vi "Build SPI Command.vi"(10 "SPI CMD FIFO Element":u64, 11 "SPI PHY Settings":T2={"Divide Value"=20, "Transfer Length (bits)"=32, "CS Asserted Polarity"=FALSE, "Clock Polarity (CPOL)"=FALSE, "Clock Phase (CPHA)"=FALSE, "Lengthen MISO Setup"=FALSE, "Direction Change Bit"=0, "MOSI Starts as Output"=FALSE, "Tristatable MOSI"=FALSE} {"Direction Change Bit" max=64 step=1; "Transfer Length (bits)" min=1 max=64 step=1}) -> (2 "SLSC SPI Command":T1={"Chip Select"=0, "CS Bit Value/Slot #"=0, "SPI PHY Settings"={"Divide Value"=0, "Transfer Length (bits)"=1, "CS Asserted Polarity"=FALSE, "Clock Polarity (CPOL)"=FALSE, "Clock Phase (CPHA)"=FALSE, "Lengthen MISO Setup"=FALSE, "Direction Change Bit"=0, "MOSI Starts as Output"=FALSE, "Tristatable MOSI"=FALSE}, "Data to DAC"=0} {"SPI PHY Settings"."Direction Change Bit" max=64 step=1; "SPI PHY Settings"."Transfer Length (bits)" min=1 max=64 step=1}, 3 "Rack #":u8)   [LabVIEW 2014, in "SLSC FPGA Toolkit.lvlib"]
uses:
  SLSC FPGA Toolkit.lvlib
  <userlib>/_NI SPI IP/FPGA/Controllers/Public/Transfer Settings.ctl
  SLSC SPI Command.ctl
  <userlib>/_NI SPI IP/FPGA/Controllers/NI SPI IP FPGA.lvlib
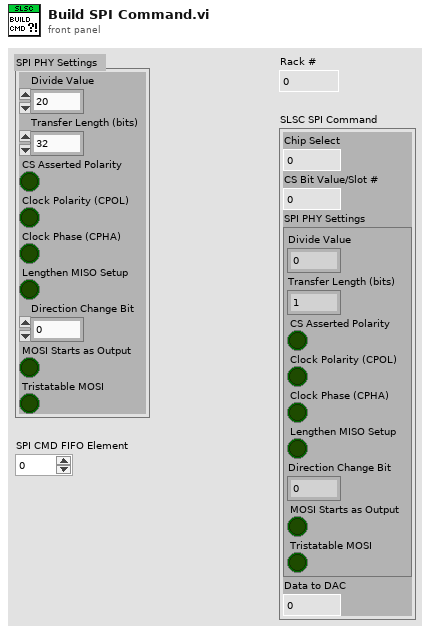
[diagram p1: front panel]
types:
  T1 = typedef "SLSC FPGA Toolkit.lvlib/SLSC SPI Command.ctl" = cluster{"Chip Select":u8, "CS Bit Value/Slot #":u8, "SPI PHY Settings":T2, "Data to DAC":u64}
  T2 = typedef "NI SPI IP FPGA.lvlib/Transfer Settings.ctl" = cluster{"Divide Value":u8, "Transfer Length (bits)":u8, "CS Asserted Polarity":bool, "Clock Polarity (CPOL)":bool, "Clock Phase (CPHA)":bool, "Lengthen MISO Setup":bool, "Direction Change Bit":u8, "MOSI Starts as Output":bool, "Tristatable MOSI":bool}
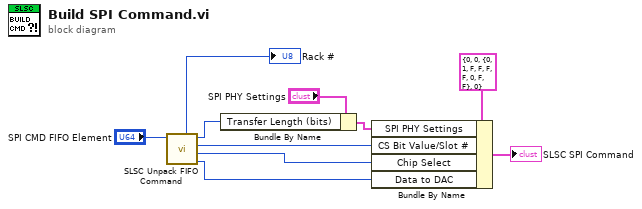
[diagram p0: block diagram]
diagram:
  n1 = call "SLSC Unpack FIFO Command.vi"("SPI CMD FIFO Element"="SPI CMD FIFO Element") -> ("Data to DAC"=w3:u64, "Chip Select"=w6:u8, "CS Bit Value/Slot #"=w7:u8, "Transfer Length"=w2:u8, "Rack #"=→"Rack #":u8)  [unwired: 6 in]
  n2 = Bundle By Name(cluster="SPI PHY Settings", "Transfer Length (bits)"=w2) -> (w4:T2)
  n3 = Bundle By Name(cluster=T1 {"Chip Select"=0, "CS Bit Value/Slot #"=0, "SPI PHY Settings"={"Divide Value"=0, "Transfer Length (bits)"=1, "CS Asserted Polarity"=FALSE, "Clock Polarity (CPOL)"=FALSE, "Clock Phase (CPHA)"=FALSE, "Lengthen MISO Setup"=FALSE, "Direction Change Bit"=0, "MOSI Starts as Output"=FALSE, "Tristatable MOSI"=FALSE}, "Data to DAC"=0}, "SPI PHY Settings"=w4, "CS Bit Value/Slot #"=w7, "Chip Select"=w6, "Data to DAC"=w3) -> (→"SLSC SPI Command":T1)
